vi "Configure Dropout Trigger.vi"(0 "VISA resource name":refnum<visa-resource-name>, 1 "Trigger Slope (0: Rising)":u16(ring) items=["Rising", "Falling"], 2 "Trigger Source (0: Channel 1)":u16(ring) items=["Channel 1", "Channel 2", "Channel 3", "Channel 4", "External", "Line", "Ext", "Ext10"], 5 "Trigger Level (0.0 V)":dbl, 11 "error in (no error)":errorcluster, 12 "Timeout (25ns)":dbl=2.5e-08) -> (4 "VISA resource name out":refnum<visa-resource-name>, 15 "error out":errorcluster)   [LabVIEW 2015, in "LeCroy Wave Series.lvlib"]
doc: "Configures dropout trigger settings. Used primarily in single-shot applications, and usually with a pre-trigger delay, Dropout trigger can detect lost signals. The trigger is generated at the end of the timeout period following the last trigger source transition.\n\nNote: \"External\" is included for the purpose of backwards compatibility. Use EXT or EXT10 for best results."
uses:
  <instrlib>/LeCroy Wave Series/LeCroy Wave Series.lvlib
panel:
  # "Note: \"External\" is included for the purpose\nof backwards compatibility.  Use EXT or EXT10\nfor best results."
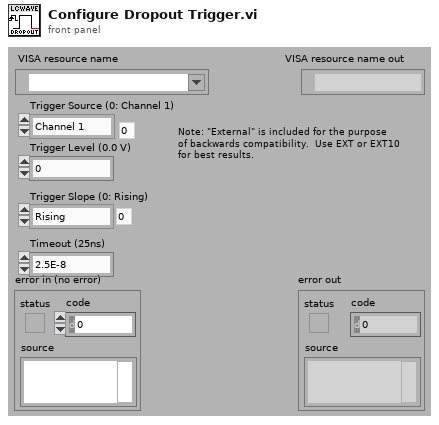
[diagram p1: front panel]
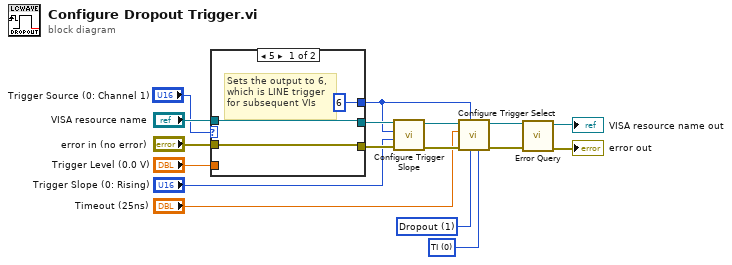
[diagram p0: block diagram]
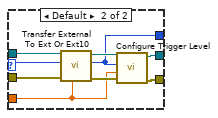
[diagram p2: hidden frame]
diagram:
  w4 = u16 0 items=["TI", "TL", "EV", "PS", "PL", "IS", "IL", "P2", "I2", "OFF"] ("Hold Type(Time)")
  w5 = u16 1 items=["Edge", "Dropout", "Glitch", "Interval", "Std", "Sng", "State Qualify", "Edge Qualify"] ("Trigger type")
  n1 = case shown="5" "Trigger Source (0: Channel 1)" {
    selector: "Trigger Source (0: Channel 1)" -> [_ w21]
    tunnel: [w19 w29] -> w17
    tunnel: [w18 w28] -> w16
    tunnel: "VISA resource name" -> [w19 w27]
    tunnel: "error in (no error)" -> [w18 w26]
    tunnel: "Trigger Level (0.0 V)" -> [_ w23]
    tunnel: [u16 6 ("Trigger Source With Ext/Ext10") w22] -> w3
    frame 5 {
      # "Sets the output to 6,\nwhich is LINE trigger\nfor subsequent VIs"
    }
    frame Default {
      n2 = call <instrlib>:"Transfer External To Ext Or Ext10.vi"("Trigger Level"=w23, "error in (no error)"=w26, "Trigger Source With External"=w21, "VISA resource name"=w27) -> ("error out"=w24:errorcluster, "Trigger Source With Ext/Ext10"=w22:u16, "VISA resource name out"=w25:refnum<visa-resource-name>)  [unwired: 5 in]
      n3 = call <instrlib>:"Configure Trigger Level.vi"("error in (no error)"=w24, "Trigger Level 1 (0.0 V)"=w23, "Channel (0: Channel 1)"=w22, "VISA resource name"=w25) -> ("error out"=w28:errorcluster, "VISA resource name out"=w29:refnum<visa-resource-name>)  [unwired: 6 in]
    }
  }
  n4 = call <instrlib>:"Configure Trigger Slope.vi"("error in (no error)"=w16, "Trigger Slope (0: Rising)"="Trigger Slope (0: Rising)", "Channel (0: Channel 1)"=w3, "VISA resource name"=w17) -> ("error out"=w13:errorcluster, "VISA resource name out"=w14:refnum<visa-resource-name>)  [unwired: 6 in]
  n5 = call <instrlib>:"Configure Trigger Select.vi"("Hold Type (0: TI)"=w4, "Trigger type"=w5, "Trigger Source (0: Channel 1)"=w3, "error in (no error)"=w13, "Hold Value 1 (4 ns)"="Timeout (25ns)", "VISA resource name"=w14) -> ("error out"=w9:errorcluster, "VISA resource name out"=w10:refnum<visa-resource-name>)  [unwired: 4 in]
  n6 = call <instrlib>:"Error Query.vi"("error in (no error)"=w9, "VISA resource name"=w10) -> ("error out"=→"error out":errorcluster, "VISA resource name out"=→"VISA resource name out":refnum<visa-resource-name>)  [unwired: 6 in, 2 out]
